vi "Read adjacency list.vi"(11 "DAG in":refnum<class "DAG.lvclass">) -> (2 "adjacency list":cluster{"edge list":i32[]}[](array[cluster]), 3 "DAG out":refnum<class "DAG.lvclass">)   [LabVIEW 2014, in "DAG.lvclass"]
uses:
  DAG.lvclass
  DAG.lvclass/DAG.ctl
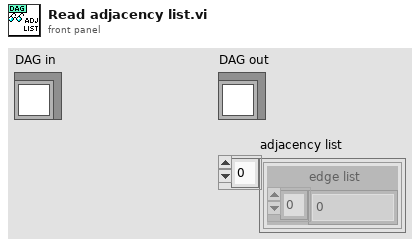
[diagram p1: front panel]
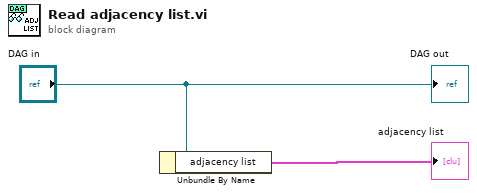
[diagram p0: block diagram]
diagram:
  n1 = Unbundle By Name("DAG in") -> ("adjacency list"=→"adjacency list":cluster{"edge list":i32[]}[])
  "DAG out" <- "DAG in"
